vi "第三版系统PID.vi"() -> ()   [LabVIEW 2015]
uses:
  <userlib>/iDAQ/iDAQ LIBs/IO Channels/AI/AI Channel.xctl
  <userlib>/iDAQ/iDAQ LIBs/IO Channels/AO/AO Channel.xctl
  <userlib>/iDAQ/iDAQ LIBs/Private/Creat/AO/iDAQ Create Channel (AO-Voltage-Basic).vi
  <userlib>/iDAQ/iDAQ LIBs/Private/Creat/AI/iDAQ Create Channel (AI-Volatge-Basic).vi
  <userlib>/iDAQ/iDAQ LIBs/Private/Read/AI/iDAQ Read (Analog DBL 1Chan 1Samp).vi
  <userlib>/iDAQ/iDAQ LIBs/Private/Write/AO/iDAQ Write (Analog DBL 1Chan 1Samp).vi
  <vilib>/Utility/file.llb/Read Delimited Spreadsheet (string).vi
panel:
  in  "越界保护(超出预警值)":bool=TRUE
  in  "实时/历史液位状态显示":enum32{"实时数据", "历史数据"}(tab)
  out "实时液位状态显示(cm)":cluster{"initial PV":dbl, "SP:":dbl, dbl, dbl}(graph)
  out "阀门输出(%)":dbl(graph)
  in  "加载历史数据":bool
  in  "历史数据路径":path=path "E:/labview project/课程设计/第三版程序/data_store/data.txt"
  out "历史液位状态显示(cm)":cluster{dbl[], dbl[]}[](graph)
  in  "PID默认参数":u16(ring) items=["一阶T1=10s", "一阶T1=50s", "一阶T1=100s", "二阶T1=10sT2=50s", "二阶T1=50sT2=50s", "二阶T1=100sT2=50s"]
  in  "控制周期 (s)":dbl=0.05
  in  "滤波数量":dbl=5.0
  in  "采样数量":dbl=25.0
  out "蓄水箱":u8(slide)=100 caption="Slide" scale=0.1..100.0
  out "手动模式":bool
  out "自动模式":bool
  in  "手动/自动切换":bool
  out "液位下限":bool
  out "液位上限":bool
  in  "液位预警值":cluster{dbl, dbl}(slide)={2.0, 28.0} scale=0.0..30.0
  in  "设定值(cm)：":dbl(slide)=10.0 min=0.0 max=0.0 scale=0.0..30.0
  in  "阀门开度(%)：":dbl(slide) scale=0.0..100.0
  out "实际值(cm)：":dbl(slide) scale=0.0..30.0
  out "自定义":bool
  out "默认":bool
  in  "自定义/默认":bool
  out "微分时间 (Td, min)":dbl
  out "积分时间 (Ti, min)":dbl
  out "比例系数(Kp)":dbl
  in  "数据存储":bool
  in  "实时数据存储路径":path=path "E:/labview project/课程设计/第三版程序/data_store/data.txt"
  in  "PID参数设置":T1={"比例系数(Kp)"=56.0, "积分时间 (Ti, min)"=23.0, "微分时间 (Td, min)"=1.0} {"微分时间 (Td, min)" min=0.0 format="%.3f"; "积分时间 (Ti, min)" min=0.0 format="%.3f"; "比例系数(Kp)" min=0.0 format="%.3f"}
  in  "AO Channel":string(xcontrol)="Dev1/ao0\r\n"
  in  "AI Channel":string(xcontrol)="Dev1/ai0\r\n"
  in  "Stop":bool
  # "基于LabVIEW的自动液位控制系统"
  # "LabVIEW控制面板"
  # "iDAQ-USB-6009采集卡"
  # "调节阀"
  # "控制水箱液位"
  # "PID自定义参数"
  # "控制水箱"
  # "水流方向"
  # "蓄水箱"
  # "循环水泵"
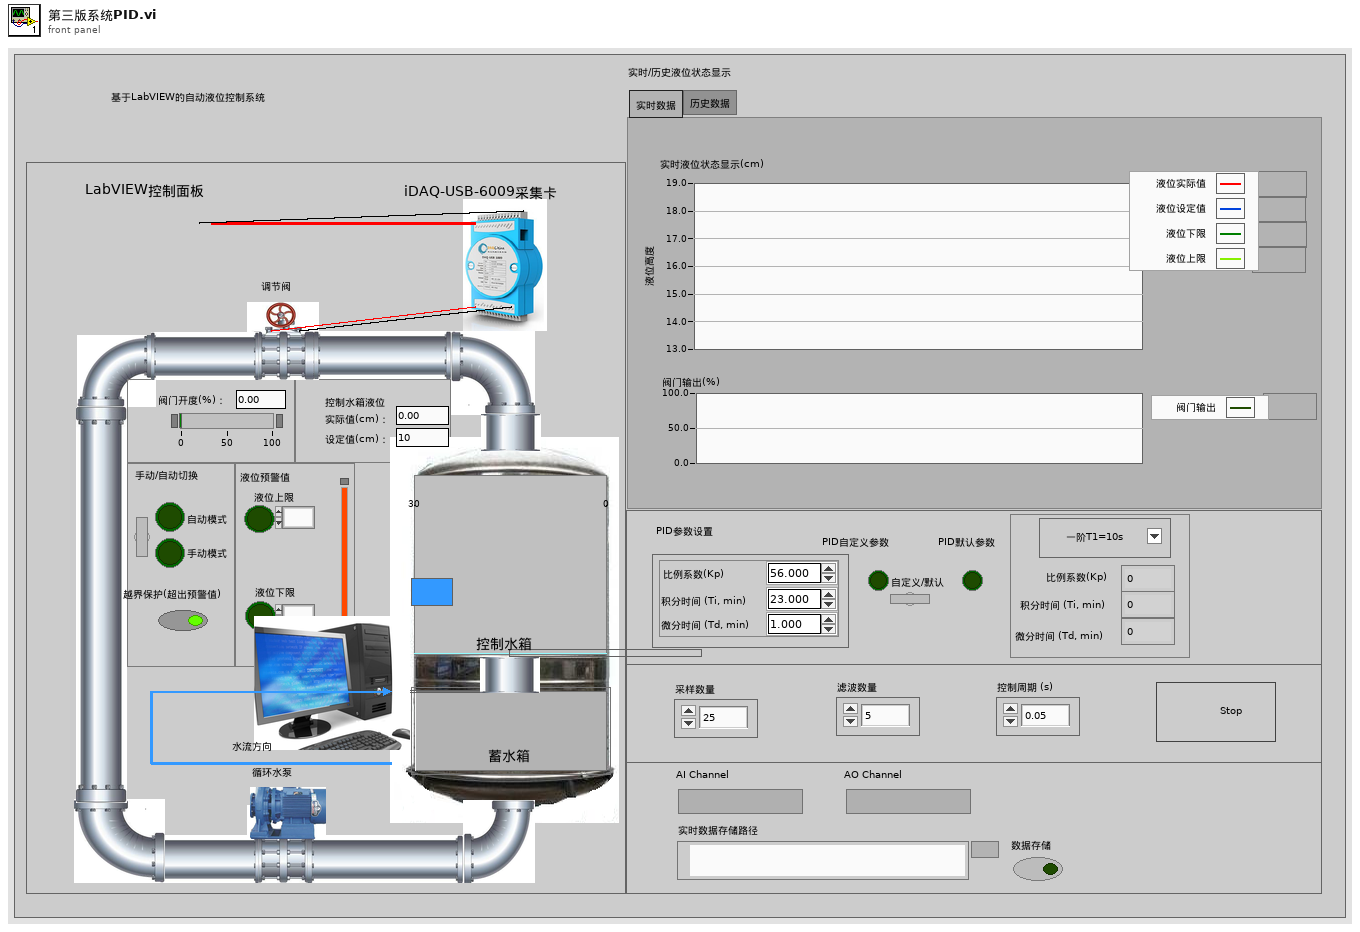
[diagram p1: front panel]
types:
  T1 = cluster{"比例系数(Kp)":dbl, "积分时间 (Ti, min)":dbl, "微分时间 (Td, min)":dbl}
  T2 = enum16{"open", "replace", "create", "open or create", "replace or create", "replace or create with confirmation"}
  T3 = typedef "设定值.ctl" = dbl
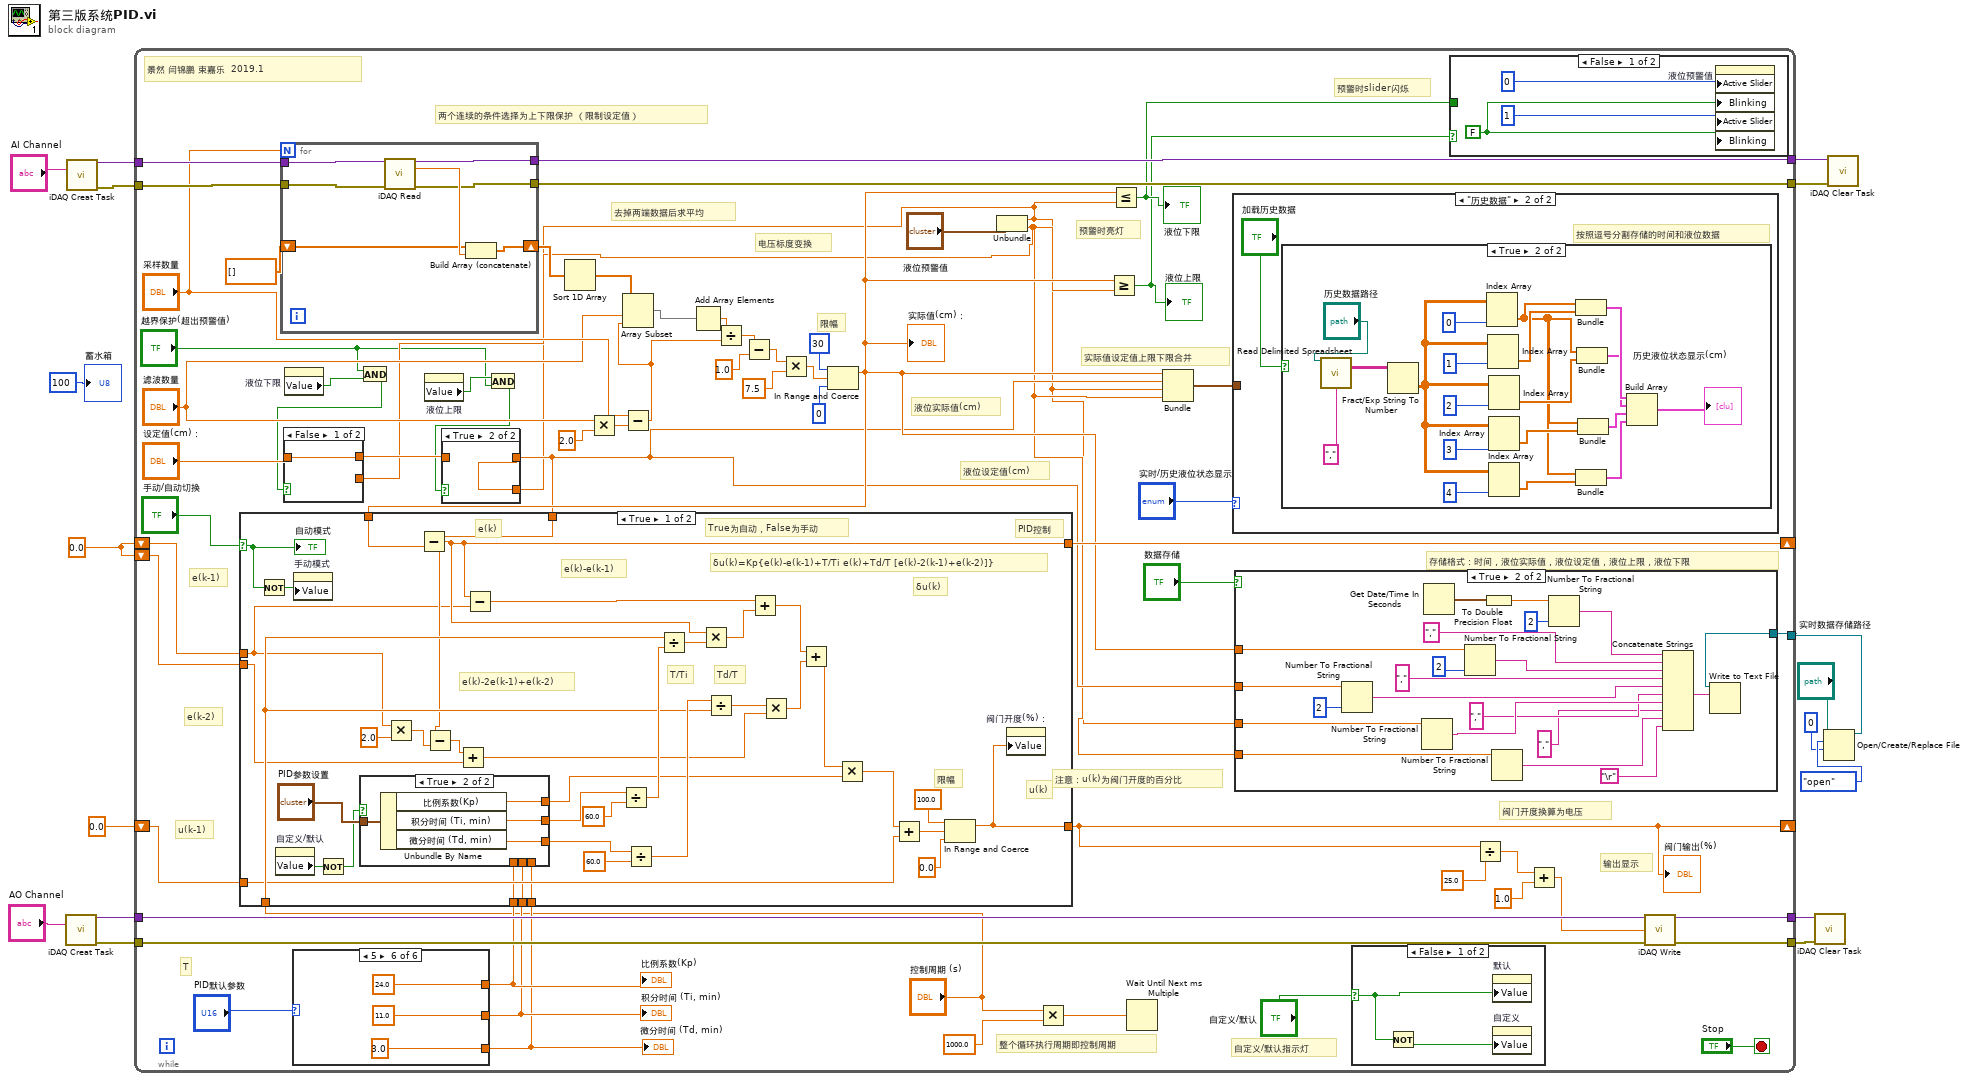
[diagram p0: block diagram]
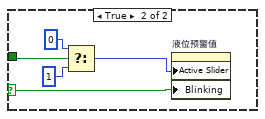
[diagram p4: hidden frame]
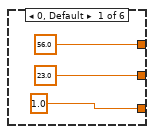
[diagram p5: hidden frame]
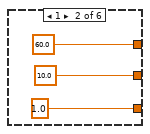
[diagram p6: hidden frame]
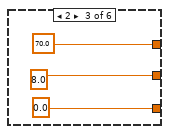
[diagram p7: hidden frame]
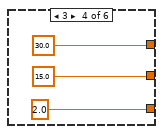
[diagram p8: hidden frame]
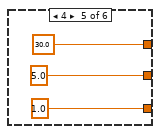
[diagram p9: hidden frame]
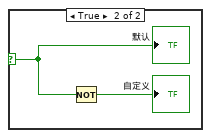
[diagram p10: hidden frame]
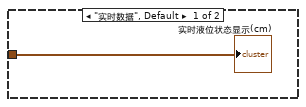
[diagram p11: hidden frame]
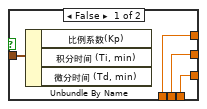
[diagram p14: hidden frame]
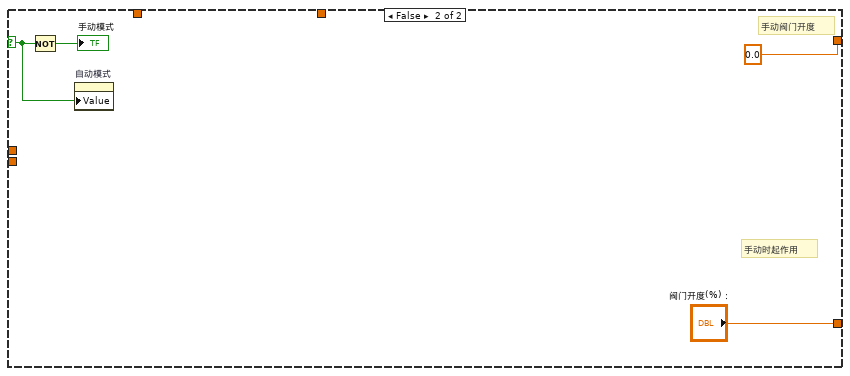
[diagram p15: hidden frame]
diagram:
  w7 = T3 0.0 ("设定值：")
  n1 = call-poly <userlib>:"iDAQ Creat Task.vi"("AO Channel"="AO Channel") -> ("Task Out"=w13:variant, "error out"=w12:errorcluster)  [unwired: 13 in]
  n2 = call-poly <userlib>:"iDAQ Creat Task.vi"("AI Channel"="AI Channel") -> ("Task Out"=w16:variant, "error out"=w15:errorcluster)  [unwired: 13 in]
  n3 = Open/Create/Replace File(file path (use dialog)="实时数据存储路径", operation (0:open)=T2."open", access (0:read/write)=0) -> (refnum out=w1:refnum<file>)  [unwired: 3 in, 2 out]
  n4 = while {
    tunnel: w16 -> [w60]
    tunnel: w15 -> [w59]
    tunnel: w13 -> [w58]
    tunnel: w12 -> [w57]
    tunnel: [w55] -> w11
    tunnel: [w54] -> w10
    tunnel: [w53] -> w9
    tunnel: [w52] -> w8
    shift-right: [w51] -> _
    shift-left: w7 -> [w48]
    shift-left: w7 -> [w50]
    shift-right: [w18] -> _
    shift-left: T3 0.0 ("设定值：") -> [w49]
    tunnel: w1 -> [w44]
    stop <- "Stop" stop-if-true
    # "景然 闫锦鹏 束嘉乐  2019.1"
    # "预警时slider闪烁"
    # "两个连续的条件选择为上下限保护 （限制设定值）"
    # "预警时亮灯"
    # "实际值设定值上限下限合并"
    # "自定义/默认指示灯"
    # "去掉两端数据后求平均"
    # "限幅"
    # "存储格式：时间，液位实际值，液位设定值，液位上限，液位下限"
    # "液位实际值(cm)"
    # "电压标度变换"
    # "整个循环执行周期即控制周期"
    # "液位设定值(cm)"
    # "阀门开度换算为电压"
    # "输出显示"
    # "注意：u(k)为阀门开度的百分比"
    # "u(k-1)"
    # "T"
    # "e(k-2)"
    # "e(k-1)"
    n5 = for {
      N: "采样数量" -> [_]
      shift-right: [w212] -> w61
      shift-left: dbl[] [] -> [w210]
      tunnel: w60 -> [w209]
      tunnel: w59 -> [w208]
      tunnel: [w207] -> w53
      tunnel: [w206] -> w52
      n6 = call-poly <userlib>:"iDAQ Read.vi"("Task In"=w209, "error in (no error)"=w208) -> ("Task Out"=w207:variant, "Data"=w211:dbl, "error out"=w206:errorcluster)  [unwired: 11 in]
      n7 = Build Array (concatenate)(w210, w211) -> (w212:dbl[])
    }
    n8 = property on="液位下限" class="Bool (strict)"() -> ("Value"=w25:bool)  [unwired: 2 in, 2 out]
    n9 = case shown="5" "PID默认参数" {
      tunnel: [56.0 60.0 70.0 30.0 30.0 24.0] -> w38
      tunnel: [23.0 10.0 8.0 15.0 5.0 11.0] -> w37
      tunnel: [1.0 1.0 0.0 2.0 1.0 3.0] -> w36
      frame 0, Default {
      }
      frame 1 {
      }
      frame 2 {
      }
      frame 3 {
      }
      frame 4 {
      }
      frame 5 {
      }
    }
    "比例系数(Kp)" <- w38
    "积分时间 (Ti, min)" <- w37
    "微分时间 (Td, min)" <- w36
    n10 = And(x="越界保护(超出预警值)", y=w25) -> (x .and. y?=w24:bool)
    n11 = property on="液位上限" class="Bool (strict)"() -> ("Value"=w22:bool)  [unwired: 2 in, 2 out]
    n12 = And(x=w22, y="越界保护(超出预警值)") -> (x .and. y?=w23:bool)
    n13 = Sort 1D Array(array=w61) -> (sorted array=w62:dbl[])
    n14 = Multiply(x="滤波数量", y=2.0) -> (x*y=w65:dbl)
    n15 = Subtract(x="采样数量", y=w65) -> (x-y=w68:dbl)
    n16 = Array Subset(array=w62, index="滤波数量", length=w68) -> (w66:dbl[])
    n17 = Add Array Elements(numeric array=w66) -> (sum=w67:dbl)
    n18 = Divide(x=w67, y=w68) -> (x/y=w69:dbl)
    n19 = Subtract(x=w69, y=1.0) -> (x-y=w71:dbl)
    n20 = Multiply(x=w71, y=7.5) -> (x*y=w41:dbl)
    n21 = In Range and Coerce(upper limit=30, x=w41, lower limit=0) -> (coerced(x)=w40:dbl)  [unwired: 1 out]
    "实际值(cm)：" <- w40
    n22 = Unbundle("液位预警值") -> (w20:dbl, w21:dbl)
    n23 = case shown="False" w24 {
      tunnel: "设定值(cm)：" -> [w82 _]
      tunnel: [w82 w83] -> w28
      tunnel: w21 -> [_ w83]
      frame False {
      }
      frame True {
      }
    }
    n24 = case shown="True" w23 {
      tunnel: [w80 w81] -> w27
      tunnel: w28 -> [w80 _]
      tunnel: w20 -> [_ w81]
      frame False {
      }
      frame True {
      }
    }
    n25 = case shown="True" "手动/自动切换" {
      selector: "手动/自动切换" -> [w166 w203]
      tunnel: w27 -> [w192 _]
      tunnel: "控制周期 (s)" -> [w184 _]
      tunnel: [w162 "阀门开度(%)："] -> w18
      tunnel: w40 -> [w191 _]
      tunnel: [w181 T3 0.0 ("设定值：")] -> w51
      tunnel: w48 -> [w161 _]
      tunnel: w50 -> [w178 _]
      tunnel: w49 -> [w169 _]
      tunnel: w38 -> [w158 _]
      tunnel: w37 -> [w160 _]
      tunnel: w36 -> [w159 _]
      frame True {
        # "PID控制"
        # "δu(k)=Kp{e(k)-e(k-1)+T/Ti e(k)+Td/T [e(k)-2(k-1)+e(k-2)]}"
        # "限幅"
        # "True为自动，False为手动"
        # "e(k)"
        # "u(k)"
        # "δu(k)"
        # "e(k)-2e(k-1)+e(k-2)"
        # "Td/T"
        # "T/Ti"
        # "e(k)-e(k-1)"
        n26 = Not(x=w166) -> (.not. x?=w167:bool)
        n27 = property on="自定义/默认" class="Bool (strict)"() -> ("Value"=w157:bool)  [unwired: 2 in, 2 out]
        n28 = property on="手动模式" class="Bool (strict)"("Value"=w167) -> ()  [unwired: 2 in, 2 out]
        n29 = Not(x=w157) -> (.not. x?=w156:bool)
        n30 = case shown="True" w156 {
          tunnel: "PID参数设置" -> [w197 w201]
          tunnel: [w196 w200] -> w190
          tunnel: [w195 w199] -> w188
          tunnel: [w194 w198] -> w170
          tunnel: w160 -> [w196 _]
          tunnel: w159 -> [w195 _]
          tunnel: w158 -> [w194 _]
          frame False {
            n31 = Unbundle By Name(w197) -> ()  [unwired: 3 out]
          }
          frame True {
            n32 = Unbundle By Name(w201) -> ("比例系数(Kp)"=w198:dbl, "积分时间 (Ti, min)"=w200:dbl, "微分时间 (Td, min)"=w199:dbl)
          }
        }
        n33 = Multiply(x=w161, y=2.0) -> (x*y=w180:T3)
        n34 = Subtract(x=w192, y=w191) -> (x-y=w181:dbl)
        n35 = Subtract(x=w181, y=w180) -> (x-y=w179:T3)
        n36 = Add(x=w179, y=w178) -> (x+y=w176:T3)
        n37 = Subtract(x=w181, y=w161) -> (x-y=w175:T3)
        n38 = Divide(x=w190, y=60.0) -> (x/y=w186:dbl)
        n39 = Divide(x=w188, y=60.0 ("x")) -> (x/y=w185:dbl)
        n40 = Divide(x=w184, y=w186) -> (x/y=w183:dbl)
        n41 = Multiply(x=w181, y=w183) -> (x*y=w174:dbl)
        n42 = Divide(x=w185, y=w184) -> (x/y=w177:dbl)
        n43 = Add(x=w175, y=w174) -> (x+y=w173:T3)
        n44 = Multiply(x=w177, y=w176) -> (x*y=w172:T3)
        n45 = Add(x=w173, y=w172) -> (x+y=w171:T3)
        n46 = Multiply(x=w171, y=w170) -> (x*y=w168:T3)
        n47 = Add(x=w168, y=w169) -> (x+y=w165:T3)
        n48 = In Range and Coerce(upper limit=T3 100.0 ("lower limit"), x=w165, lower limit=T3 0.0) -> (coerced(x)=w162:T3)  [unwired: 1 out]
        n49 = property on="阀门开度(%)：" class="Slide (strict)"("Value"=w162) -> ()  [unwired: 2 in, 2 out]
        "自动模式" <- w166
      }
      frame False {
        # "手动阀门开度"
        # "手动时起作用"
        n50 = Not(x=w203) -> (.not. x?=→"手动模式":bool)
        n51 = property on="自动模式" class="Bool (strict)"("Value"=w203) -> ()  [unwired: 2 in, 2 out]
      }
    }
    "阀门输出(%)" <- w18
    n52 = Multiply(x="控制周期 (s)", y=1000.0) -> (x*y=w74:dbl)
    n53 = Greater Or Equal?(x=w40, y=w21) -> (x >= y?=w34:bool)
    "液位上限" <- w34
    n54 = Less Or Equal?(x=w40, y=w20) -> (x <= y?=w35:bool)
    "液位下限" <- w35
    n55 = Wait Until Next ms Multiple(millisecond multiple=w74) -> ()  [unwired: 1 out]
    n56 = Bundle(w40, "设定值(cm)："=w27, w20, w21) -> (w45:cluster{dbl, "设定值(cm)：":dbl, dbl, dbl})  [unwired: 1 in]
    n57 = case shown="\"历史数据\"" "实时/历史液位状态显示" {
      tunnel: w45 -> [w114 _]
      frame "实时数据", Default {
        "实时液位状态显示(cm)" <- w114
      }
      frame "历史数据" {
        # "按照逗号分割存储的时间和液位数据"
        n58 = case shown="True" "加载历史数据" {
          frame False {
          }
          frame True {
            n59 = call-poly <vilib>:"Read Delimited Spreadsheet.vi"("file path (dialog if empty)"="历史数据路径", "delimiter (\\t)"=",") -> ("all rows"=w129:string[][])  [unwired: 8 in, 5 out]
            n60 = Fract/Exp String To Number(string=w129) -> (number=w120:dbl[][])  [unwired: 3 in, 1 out]
            n61 = Index Array(array=w120, index (col)=0) -> (element=w116:dbl[])  [unwired: 1 in]
            n62 = Index Array(array=w120, index (col)=1) -> (element=w132:dbl[])  [unwired: 1 in]
            n63 = Index Array(array=w120, index (col)=2) -> (element=w125:dbl[])  [unwired: 1 in]
            n64 = Index Array(array=w120, index (col)=3) -> (element=w119:dbl[])  [unwired: 1 in]
            n65 = Index Array(array=w120, index (col)=4) -> (element=w121:dbl[])  [unwired: 1 in]
            n66 = Bundle(w116, w132) -> (w133:cluster{dbl[], dbl[]})  [unwired: 1 in]
            n67 = Bundle(w116, w121) -> (w118:cluster{dbl[], dbl[]})  [unwired: 1 in]
            n68 = Bundle(w116, w125) -> (w124:cluster{dbl[], dbl[]})  [unwired: 1 in]
            n69 = Bundle(w116, w119) -> (w117:cluster{dbl[], dbl[]})  [unwired: 1 in]
            n70 = Build Array(w133, w124, w117, w118) -> (→"历史液位状态显示(cm)":cluster{dbl[], dbl[]}[])
          }
        }
      }
    }
    n71 = case shown="True" "数据存储" {
      tunnel: w40 -> [_ w147]
      tunnel: w44 -> [_ w146]
      tunnel: w27 -> [_ w142]
      tunnel: w20 -> [_ w141]
      tunnel: w21 -> [_ w140]
      frame False {
      }
      frame True {
        n72 = Number To Fractional String(number=w142, precision (6)=i16 2) -> (F-format string=w143:string)  [unwired: 2 in]
        n73 = Number To Fractional String(number=w141) -> (F-format string=w139:string)  [unwired: 3 in]
        n74 = Get Date/Time In Seconds() -> (seconds since 1Jan1904=w155:timestamp)
        n75 = Number To Fractional String(number=w147, precision (6)=i16 2) -> (F-format string=w149:string)  [unwired: 2 in]
        n76 = To Double Precision Float(number=w155) -> (double precision float=w154:dbl)
        n77 = Number To Fractional String(number=w140) -> (F-format string=w136:string)  [unwired: 3 in]
        n78 = Number To Fractional String(number=w154, precision (6)=i16 2) -> (F-format string=w151:string)  [unwired: 2 in]
        n79 = Concatenate Strings(w151, ",", w149, ",", w143, ",", w139, ",", w136, "\r") -> (w148:string)
        n80 = Write to Text File(file (use dialog)=w146, text=w148) -> ()  [unwired: 2 in, 3 out]
      }
    }
    n81 = case shown="False" "自定义/默认" {
      selector: "自定义/默认" -> [w111 w112]
      frame False {
        n82 = Not(x=w111) -> (.not. x?=w110:bool)
        n83 = property on="默认" class="Bool (strict)"("Value"=w111) -> ()  [unwired: 2 in, 2 out]
        n84 = property on="自定义" class="Bool (strict)"("Value"=w110) -> ()  [unwired: 2 in, 2 out]
      }
      frame True {
        n85 = Not(x=w112) -> (.not. x?=→"自定义":bool)
        "默认" <- w112
      }
    }
    n86 = case shown="False" w34 {
      selector: w34 -> [_ w87]
      tunnel: w35 -> [_ w89]
      frame False {
        w86 = FALSE ("Blinking")
        n87 = property on="液位预警值" class="Slide (strict)"("Active Slider"=0, "Blinking"=w86, "Active Slider"=1, "Blinking"=w86) -> ()  [unwired: 2 in, 2 out]
      }
      frame True {
        n88 = Select(t=0 ("Active Slider"), s=w89, f=1 ("Active Slider")) -> (s? t:f=w88:i32)
        n89 = property on="液位预警值" class="Slide (strict)"("Active Slider"=w88, "Blinking"=w87) -> ()  [unwired: 2 in, 2 out]
      }
    }
    n90 = Divide(x=w18, y=25.0 ("x/y")) -> (x/y=w78:T3)
    n91 = Add(x=w78, y=1.0) -> (x+y=w47:T3)
    n92 = call-poly <userlib>:"iDAQ Write.vi"("Task In"=w58, "data"=w47, "error in (no error)"=w57) -> ("Task Out"=w55:variant, "error out"=w54:errorcluster)  [unwired: 11 in]
  }
  n93 = call <userlib>:"iDAQ Clear Task.vi"("error in (no error)"=w10, "Task In"=w11) -> ()  [unwired: 9 in, 1 out]
  n94 = call <userlib>:"iDAQ Clear Task.vi"("error in (no error)"=w8, "Task In"=w9) -> ()  [unwired: 9 in, 1 out]
  "蓄水箱" <- 100
